vi "Read TopVI Tag.vi"(8 "error in":errorcluster, 10 "Project Reference":refnum<vi>) -> (0 "error out":errorcluster, 2 "TopVI Tag":string, 3 "TopVI Path":path)   [LabVIEW 2020]
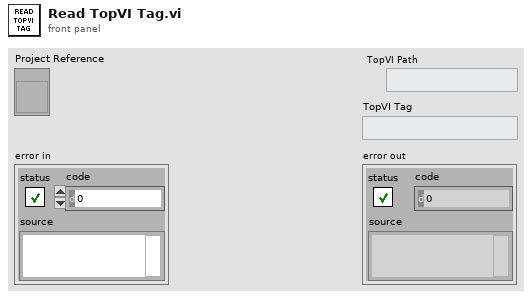
[diagram p1: front panel]
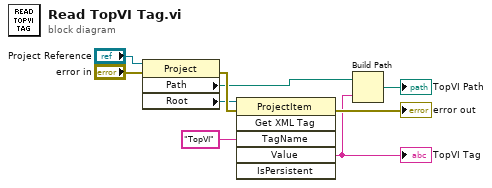
[diagram p0: block diagram]
diagram:
  n1 = property class="Project"(reference="Project Reference", error in="error in") -> (error out=w9:errorcluster, "Path"=w5:path, "Root"=w4:refnum<vi>)  [unwired: 1 out]
  n2 = invoke class="ProjectItem" method="Get XML Tag"(reference=w4, error in=w9, "TagName"="TopVI" ("Tag Name")) -> (error out=→"error out":errorcluster, "Value"=w2:string)  [unwired: 3 in, 4 out]
  "TopVI Tag" <- w2
  n3 = Build Path(base path=w5, name or relative path=w2) -> (appended path=→"TopVI Path":path)
